vi "校准泵控制.vi"(8 "错误输入（无错误）":errorcluster, 9 "摄氏度":u16, 10 "偏心轮":u16, 11 "枚举":enum16{"进水样", "进纯水", "排液", "加热", "停止"}(ring)) -> (0 "错误输出":errorcluster)   [LabVIEW 2016, in "斯坦道CODMn新电路板.lvlib"]
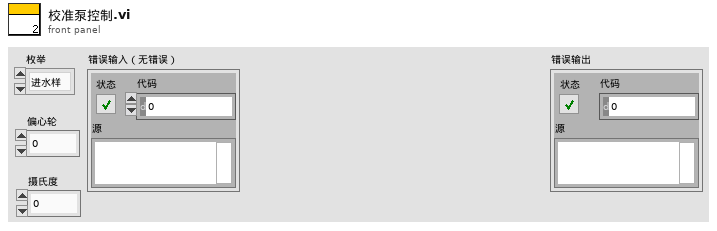
[diagram p1: front panel]
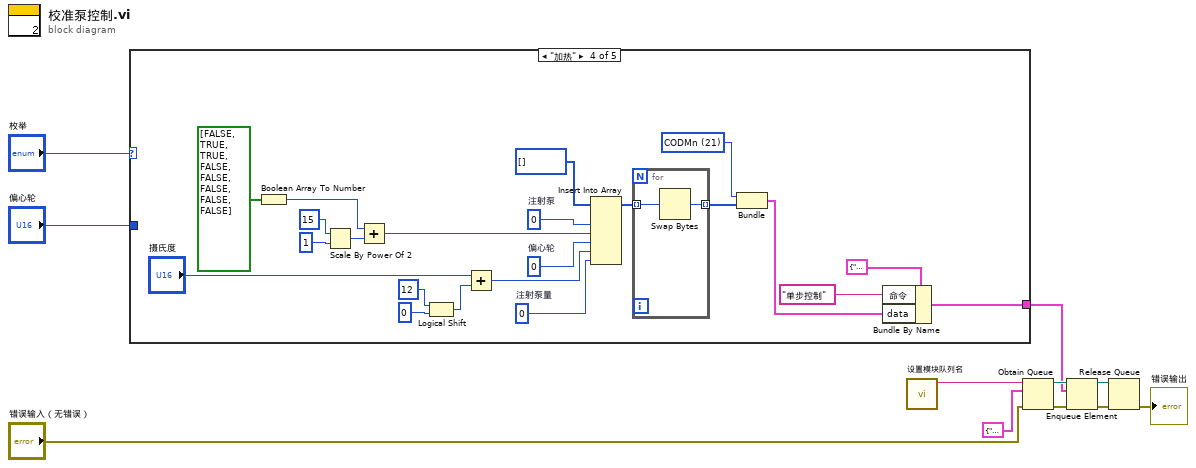
[diagram p0: block diagram]
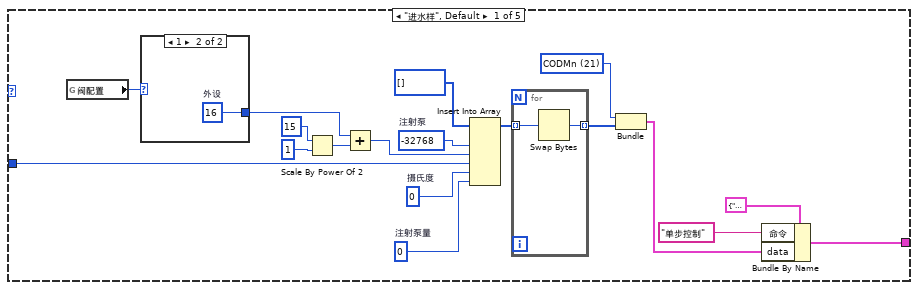
[diagram p2: hidden frame]
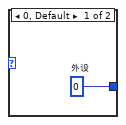
[diagram p3: hidden frame]
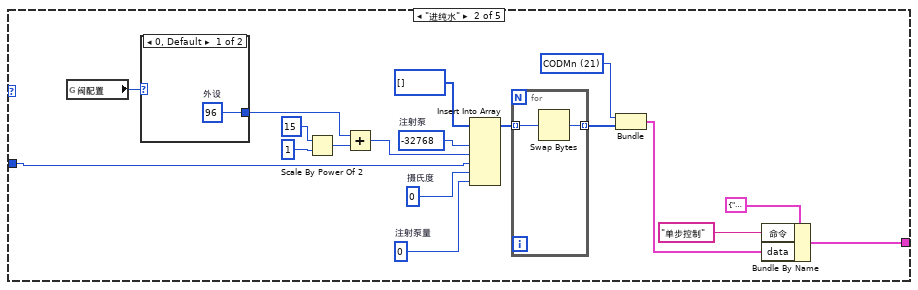
[diagram p4: hidden frame]
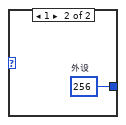
[diagram p5: hidden frame]
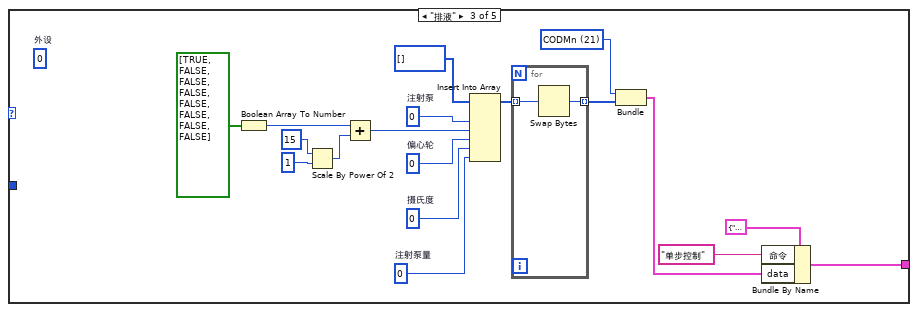
[diagram p6: hidden frame]
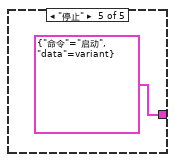
[diagram p7: hidden frame]
diagram:
  n1 = case shown="\"加热\"" "枚举" {
    tunnel: [w20 w41 w62 w87 cluster{"命令":string, "data":variant} {"命令"="启动", "data"=variant(cluster{"站号":u16, "控制命令":u16[]} {"站号"=21, "控制命令"=[2816]})} ("启动命令")] -> w5
    tunnel: "偏心轮" -> [w18 w39 _ _ _]
    frame "进水样", Default {
      w14 = i16 -32768  # 注射泵
      w25 = u16 21 items=["CODMn"=21, "总磷"=1, "氨氮"=3] ("站号")
      w28 = u16 0  # 注射泵量
      w27 = u16 0  # 摄氏度
      n2 = global read "CODMn断电保存全局变量.vi" "阀配置"() -> (w19:u8)
      n3 = case shown="1" w19 {
        tunnel: [w30 w31] -> w13
        frame 0, Default {
          w30 = u16 0  # 外设
        }
        frame 1 {
          w31 = u16 16  # 外设
        }
      }
      n4 = Scale By Power Of 2(n=i16 15, x=u16 1 ("y")) -> (x*2^n=w15:u16)
      n5 = Add(x=w13, y=w15) -> (x+y=w12:u16)
      n6 = Insert Into Array(array=u16[] [] ("数组"), new element #1=w14, new element #2=w12, new element #3=w18, new element #4=w27, new element #5=w28) -> (w26:u16[])  [unwired: 1 in]
      n7 = for {
        tunnel: w26 -> [w33] mode=indexing
        tunnel: [w32] -> w22 mode=indexing
        n8 = Swap Bytes(anything=w33) -> (byte swapped=w32:u16)
      }
      n9 = Bundle("站号"=w25, w22) -> (w24:cluster{"站号":u16, u16[]})  [unwired: 1 in]
      n10 = Bundle By Name(cluster=cluster{"命令":string, "data":variant} {"命令"="", "data"=variant} ("元素"), "命令"="单步控制", "data"=w24) -> (w20:cluster{"命令":string, "data":variant})
    }
    frame "进纯水" {
      w46 = u16 21 items=["CODMn"=21, "总磷"=1, "氨氮"=3] ("站号")
      w49 = u16 0  # 注射泵量
      w48 = u16 0  # 摄氏度
      w50 = i16 -32768  # 注射泵
      n11 = global read "CODMn断电保存全局变量.vi" "阀配置"() -> (w40:u8)
      n12 = case shown="0, Default" w40 {
        tunnel: [w52 w53] -> w36
        frame 0, Default {
          w52 = u16 96  # 外设
        }
        frame 1 {
          w53 = u16 256  # 外设
        }
      }
      n13 = Scale By Power Of 2(n=i16 15, x=u16 1 ("y")) -> (x*2^n=w35:u16)
      n14 = Add(x=w36, y=w35) -> (x+y=w34:u16)
      n15 = Insert Into Array(array=u16[] [] ("数组"), new element #1=w50, new element #2=w34, new element #3=w39, new element #4=w48, new element #5=w49) -> (w47:u16[])  [unwired: 1 in]
      n16 = for {
        tunnel: w47 -> [w55] mode=indexing
        tunnel: [w54] -> w43 mode=indexing
        n17 = Swap Bytes(anything=w55) -> (byte swapped=w54:u16)
      }
      n18 = Bundle("站号"=w46, w43) -> (w45:cluster{"站号":u16, u16[]})  [unwired: 1 in]
      n19 = Bundle By Name(cluster=cluster{"命令":string, "data":variant} {"命令"="", "data"=variant} ("元素"), "命令"="单步控制", "data"=w45) -> (w41:cluster{"命令":string, "data":variant})
    }
    frame "排液" {
      w67 = u16 21 items=["CODMn"=21, "总磷"=1, "氨氮"=3] ("站号")
      w71 = u16 0  # 注射泵量
      w70 = u16 0  # 摄氏度
      w68 = u16 0  # 偏心轮
      (unwired) u16 0  # 外设
      w72 = u16 0  # 注射泵
      n20 = Boolean Array To Number ("布尔数组至数值转换")(Boolean array=bool[] [TRUE, FALSE, FALSE, FALSE, FALSE, FALSE, FALSE, FALSE] ("添加的数组")) -> (number=w61:u16)
      n21 = Scale By Power Of 2(n=i16 15, x=u16 1 ("y")) -> (x*2^n=w60:u16)
      n22 = Add(x=w61, y=w60) -> (x+y=w56:u16)
      n23 = Insert Into Array(array=u16[] [] ("数组"), new element #1=w72, new element #2=w56, new element #3=w68, new element #4=w70, new element #5=w71) -> (w69:u16[])  [unwired: 1 in]
      n24 = for {
        tunnel: w69 -> [w75] mode=indexing
        tunnel: [w74] -> w64 mode=indexing
        n25 = Swap Bytes(anything=w75) -> (byte swapped=w74:u16)
      }
      n26 = Bundle("站号"=w67, w64) -> (w66:cluster{"站号":u16, u16[]})  [unwired: 1 in]
      n27 = Bundle By Name(cluster=cluster{"命令":string, "data":variant} {"命令"="", "data"=variant} ("元素"), "命令"="单步控制", "data"=w66) -> (w62:cluster{"命令":string, "data":variant})
    }
    frame "加热" {
      w92 = u16 21 items=["CODMn"=21, "总磷"=1, "氨氮"=3] ("站号")
      w95 = u16 0  # 注射泵量
      w93 = u16 0  # 偏心轮
      w96 = u16 0  # 注射泵
      n28 = Boolean Array To Number ("布尔数组至数值转换")(Boolean array=bool[] [FALSE, TRUE, TRUE, FALSE, FALSE, FALSE, FALSE, FALSE] ("添加的数组")) -> (number=w81:u16)
      n29 = Scale By Power Of 2(n=i16 15, x=u16 1 ("y")) -> (x*2^n=w80:u16)
      n30 = Add(x=w81, y=w80) -> (x+y=w76:u16)
      n31 = Logical Shift(y=i16 12, x=i16 0) -> (x << y=w85:i16)
      n32 = Add(x="摄氏度", y=w85) -> (x+y=w82:u16)
      n33 = Insert Into Array(array=u16[] [] ("数组"), new element #1=w96, new element #2=w76, new element #3=w93, new element #4=w82, new element #5=w95) -> (w94:u16[])  [unwired: 1 in]
      n34 = for {
        tunnel: w94 -> [w99] mode=indexing
        tunnel: [w98] -> w89 mode=indexing
        n35 = Swap Bytes(anything=w99) -> (byte swapped=w98:u16)
      }
      n36 = Bundle("站号"=w92, w89) -> (w91:cluster{"站号":u16, u16[]})  [unwired: 1 in]
      n37 = Bundle By Name(cluster=cluster{"命令":string, "data":variant} {"命令"="", "data"=variant} ("元素"), "命令"="单步控制", "data"=w91) -> (w87:cluster{"命令":string, "data":variant})
    }
    frame "停止" {
    }
  }
  n38 = call "设置模块队列名.vi"() -> ("Msg"=w1:string)  [unwired: 11 in]
  n39 = Obtain Queue(name (unnamed)=w1, element data type=cluster{"命令":string, "data":variant} {"命令"="", "data"=variant}, error in (no error)="错误输入（无错误）") -> (queue out=w10:refnum<queue>, error out=w9:errorcluster)  [unwired: 2 in, 1 out]
  n40 = Enqueue Element(queue=w10, element=w5, error in (no error)=w9) -> (queue out=w8:refnum<queue>, error out=w7:errorcluster)  [unwired: 1 in, 1 out]
  n41 = Release Queue(queue=w8, error in (no error)=w7) -> (error out=→"错误输出":errorcluster)  [unwired: 1 in, 2 out]
